vi "Load Config.vi"(8 "error in (no error)":errorcluster, 11 "Data Logger Module in":refnum<class "Data Logger DBL Module.lvclass">) -> (0 "error out":errorcluster, 3 "Data Logger Module out":refnum<class "Data Logger DBL Module.lvclass">)   [LabVIEW 2020, in "VolatusData.lvlib" / "Data Logger DBL Module.lvclass"]
uses:
  Data Logger DBL Module.lvclass
  C:/dev/lv20CE/relink/lv-volatus/Volatus/Module/Module.lvclass
  Volatus/Module/Module.lvclass/Module.ctl
  VolatusConfig/VolatusConfigElement/VolatusConfigElement.lvclass/VolatusConfigElement.ctl
  Data Logger DBL Module.lvclass/Data Logger DBL Module.ctl
  VolatusConfig/VolatusConfigElement/Element.vi
  Volatus/Module/Module.lvclass
  VolatusConfig/VolatusConfigElement/VolatusConfigElement.lvclass
  lv-cdm/CDM-Config/Config Element/Config Element.lvclass
  C:/dev/lv20CE/relink/lv-volatus/VolatusData/Data Logger DBL Module/Data Logger DBL Module.lvclass
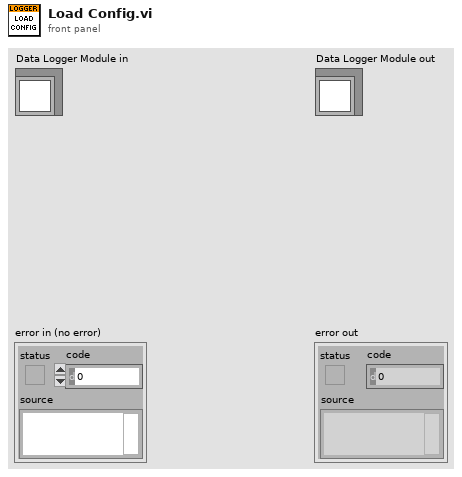
[diagram p1: front panel]
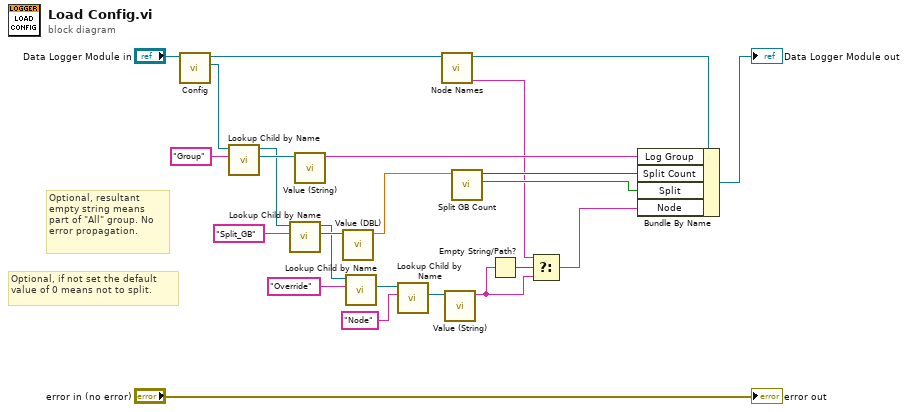
[diagram p0: block diagram]
diagram:
  # "Optional, if not set the default value of 0 means not to split."
  # "Optional, resultant empty string means part of \"All\" group. No error propagation."
  n1 = call "Config.vi"("Module in"="Data Logger Module in") -> ("Config"=w21:refnum<class "VolatusConfigElement.lvclass">, "Module out"=w22:refnum<class "Data Logger DBL Module.lvclass">)  [unwired: 9 in]
  n2 = call "Lookup Child by Name.vi"("Child Name"="Group", "VolatusConfigElement in"=w21) -> ("Child"=w19:refnum<class "Config Element.lvclass">, "VolatusConfigElement out"=w16:refnum<class "VolatusConfigElement.lvclass">)  [unwired: 6 in, 2 out]
  n3 = call "Lookup Child by Name.vi"("Child Name"="Split_GB", "VolatusConfigElement in"=w16) -> ("Child"=w14:refnum<class "Config Element.lvclass">, "VolatusConfigElement out"=w10:refnum<class "VolatusConfigElement.lvclass">)  [unwired: 6 in, 2 out]
  n4 = call "Value (String).vi"("Config Element in"=w19) -> ("String Value"=w17:string)  [unwired: 9 in, 1 out]
  n5 = call "Value (DBL).vi"("Config Element in"=w14) -> ("DBL Value"=w13:dbl)  [unwired: 9 in, 1 out]
  n6 = call "Lookup Child by Name.vi"("Child Name"="Override", "VolatusConfigElement in"=w10) -> ("Child"=w8:refnum<class "Config Element.lvclass">)  [unwired: 6 in, 3 out]
  n7 = call "Lookup Child by Name.vi"("Name"="Node", "Config Element in"=w8) -> ("Child"=w6:refnum<class "Config Element.lvclass">)  [unwired: 6 in, 3 out]
  n8 = call "Node Names.vi"("Module in"=w22) -> ("Node"=w2:string, "Module out"=w3:refnum<class "Data Logger DBL Module.lvclass">)  [unwired: 6 in, 3 out]
  n9 = call "Value (String).vi"("Config Element in"=w6) -> ("String Value"=w4:string)  [unwired: 9 in, 1 out]
  n10 = call "Split GB Count.vi"("Split GB"=w13) -> ("Split"=w11:bool, "Split Count"=w12:i32)  [unwired: 9 in]
  n11 = Empty String/Path?(string/path=w4) -> (empty?=w5:bool)
  n12 = Select(t=w2, s=w5, f=w4) -> (s? t:f=w1:string)
  n13 = Bundle By Name(cluster=w3, "Log Group"=w17, "Split Count"=w12, "Split"=w11, "Node"=w1) -> (→"Data Logger Module out":refnum<class "Data Logger DBL Module.lvclass">)
  "error out" <- "error in (no error)"
